vi "strings to line.vi"(11 "strings":string[](array[string])) -> (3 "line":T1)   [LabVIEW 2013, in "Profibus Module editor node.lvclass"]
uses:
  Profibus Module editor node.lvclass
  table line.ctl
  channel/Profibus channel.lvclass
  <vilib>/NI/Tag Bus/tag/Data Type.ctl
  permissions.ctl
  <vilib>/NI/Tag Bus/tag/tag descriptor.lvclass/tag descriptor.ctl
  channel/Profibus channel.lvclass/Profibus channel.ctl
  <vilib>/NI/Tag Bus Module Framework/channel/TBM channel.lvclass/TBM channel.ctl
  <vilib>/NI/Tag Bus/tag/write tag name.vi
  channel/Write slave.vi
  channel/Write byte.vi
  channel/Write bit.vi
  <vilib>/NI/Tag Bus Module Framework/channel/Write channel classification.vi
  <vilib>/NI/Tag Bus/tag/write data type.vi
  <vilib>/NI/Tag Bus/tag/tag descriptor.lvclass
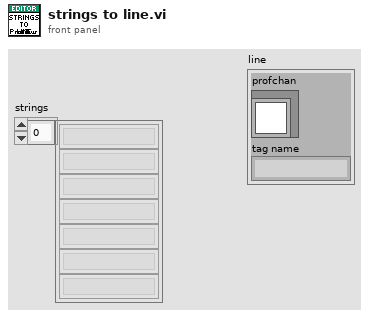
[diagram p1: front panel]
types:
  T1 = typedef "Profibus Module editor node.lvclass/table line.ctl" = cluster{"profchan":refnum<class "Profibus channel.lvclass">, "tag name":string}
  T2 = typedef "Profibus Module editor node.lvclass/permissions.ctl" = enum32{"Read from HW", "Write to HW"}
  T3 = typedef "tag bus.lvlib/tag descriptor.lvclass/Data Type.ctl" = enum16{"Double", "Single", "I64", "I32", "I16", "I8", "U64", "U32", "U16", "U8", "Boolean", "String", "Array of Double", "Array of Single", "Array of I64", "Array of I32", "Array of I16", "Array of I8", "Array of U64", "Array of U32", "Array of U16", "Array of U8", "Array of Boolean", "Array of String"}
  T4 = typedef "TBM channel.lvclass/channel classification.ctl" = enum16{"input data", "output data", "processing parameter", "processing result"}
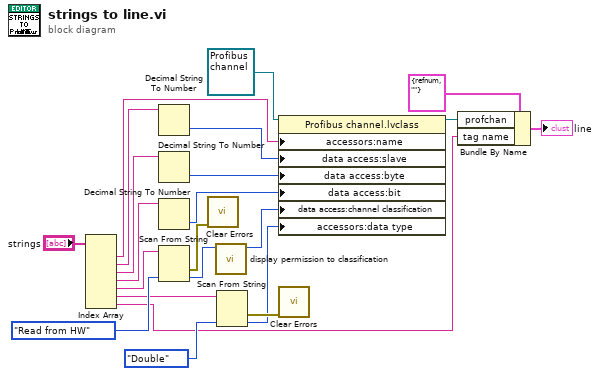
[diagram p0: block diagram]
diagram:
  n1 = Index Array(array="strings") -> (element #1=w11:string, element #2=w4:string, element #3=w5:string, element #4=w6:string, element #5=w7:string, element #6=w8:string, element #7=w9:string)  [unwired: 7 in]
  n2 = Decimal String To Number(string=w4) -> (number=w3:i32)  [unwired: 2 in, 1 out]
  n3 = Decimal String To Number(string=w5) -> (number=w2:i32)  [unwired: 2 in, 1 out]
  n4 = Decimal String To Number(string=w6) -> (number=w1:i32)  [unwired: 2 in, 1 out]
  n5 = Scan From String(input string=w7, default 1=permissions."Read from HW" ("direction")) -> (error out=w17:errorcluster, output 1=w15:T2)  [unwired: 3 in, 2 out]
  n6 = call <vilib>:"Clear Errors.vi"("error in (no error)"=w17) -> ()  [unwired: 6 in, 1 out]
  n7 = call "display permission to classification.vi"("display permissions"=w15) -> ("channel classification"=w12:T4)  [unwired: 10 in]
  n8 = Scan From String(input string=w8, default 1=Data_Type."Double" ("data type")) -> (error out=w19:errorcluster, output 1=w13:T3)  [unwired: 3 in, 2 out]
  n9 = property class="Profibus channel.lvclass"(reference=refnum<class "Profibus channel.lvclass"> refnum ("Profibus channel.lvclass"), "accessors:name"=w11, "data access:slave"=w3, "data access:byte"=w2, "data access:bit"=w1, "data access:channel classification"=w12, "accessors:data type"=w13) -> (reference out=w14:refnum<class "Profibus channel.lvclass">)  [unwired: 1 in, 1 out]
  n10 = call <vilib>:"Clear Errors.vi"("error in (no error)"=w19) -> ()  [unwired: 6 in, 1 out]
  n11 = Bundle By Name(cluster=T1 {"profchan"=refnum, "tag name"=""} ("line"), "profchan"=w14, "tag name"=w9) -> (→"line":T1)
